vi "Time_Date String To Stamp.vi"(9 "Split":string="/", 10 "Data String":string) -> (2 "Time Stamp":timestamp)   [LabVIEW 2016]
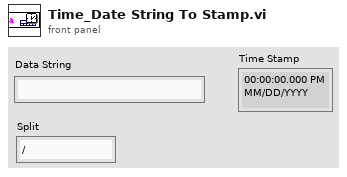
[diagram p1: front panel]
types:
  T1 = typedef "LVDateTimeRec.ctl" = cluster{"秒数的小数部分":dbl, "秒":i32, "分":i32, "小时":i32, "日":i32, "月":i32, "年":i32, "天数（周）":i32, "天数（年）":i32, "DST":i32}
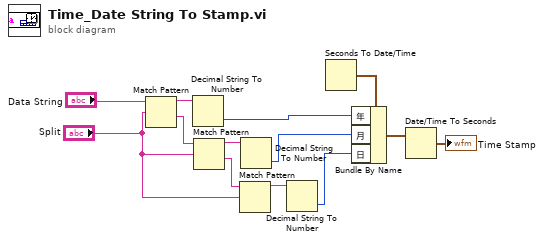
[diagram p0: block diagram]
diagram:
  n1 = Match Pattern(string="Data String", regular expression="Split") -> (before substring=w10:string, after substring=w8:string)  [unwired: 1 in, 2 out]
  n2 = Decimal String To Number(string=w10) -> (number=w9:i32)  [unwired: 2 in, 1 out]
  n3 = Match Pattern(string=w8, regular expression="Split") -> (before substring=w7:string, after substring=w3:string)  [unwired: 1 in, 2 out]
  n4 = Match Pattern(string=w3, regular expression="Split") -> (before substring=w5:string)  [unwired: 1 in, 3 out]
  n5 = Decimal String To Number(string=w7) -> (number=w6:i32)  [unwired: 2 in, 1 out]
  n6 = Decimal String To Number(string=w5) -> (number=w2:i32)  [unwired: 2 in, 1 out]
  n7 = Seconds To Date/Time() -> (date time rec=w13:T1)  [unwired: 2 in]
  n8 = Bundle By Name(cluster=w13, "年"=w9, "月"=w6, "日"=w2) -> (w12:T1)
  n9 = Date/Time To Seconds(2:w12) -> (0:→"Time Stamp":timestamp)  [unwired: 1 in]
